vi "Configure Sweep Mode.vi"(5 "Return Time (1s)":dbl=1.0 format="%#.6g", 7 "Hold Time (0 s)":dbl format="%#.6g", 8 "error in (no error)":errorcluster, 9 "Sweep Mode (0: Repeated)":u16(ring) items=["Repeated", "Triggered"], 10 "Channel (0: Channel 1)":u16(ring) items=["Channel 1", "Channel 2"], 11 "VISA resource name":refnum<visa-resource-name>) -> (0 "error out":errorcluster, 3 "VISA resource name out":refnum<visa-resource-name>)   [LabVIEW 2015, in "Tektronix AFG 3000 Series.lvlib"]
doc: "Configures the sweep mode. The VI decides whether the function generator produces a sweep when it receives a trigger or continuous sweep at a rate spedified by sweep time, hold time and return time."
uses:
  Tektronix AFG 3000 Series.lvlib
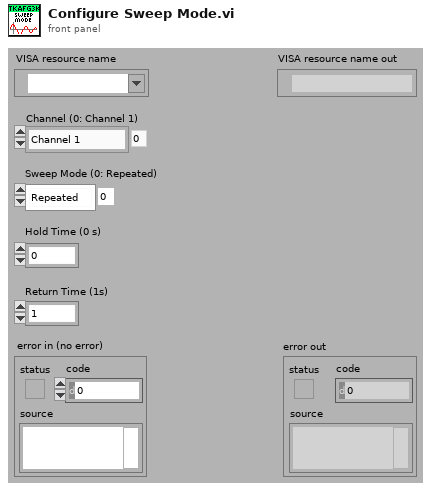
[diagram p1: front panel]
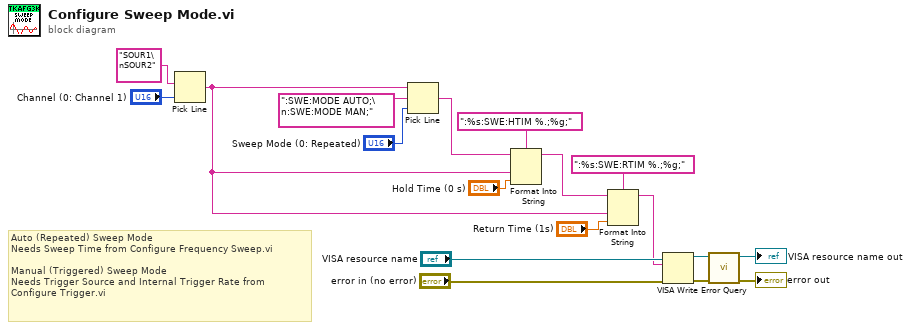
[diagram p0: block diagram]
diagram:
  # "Auto (Repeated) Sweep Mode\nNeeds Sweep Time from Configure Frequency Sweep.vi\n\nManual (Triggered) Sweep Mode\nNeeds Trigger Source and Internal Trigger Rate from\nConfigure Trigger.vi"
  n1 = Pick Line(multi-line string="SOUR1\nSOUR2" ("string (\"\")"), line index="Channel (0: Channel 1)") -> (output string=w2:string)  [unwired: 1 in]
  n2 = Pick Line(string ("")=w2, multi-line string=":SWE:MODE AUTO;\n:SWE:MODE MAN;", line index="Sweep Mode (0: Repeated)") -> (output string=w6:string)
  n3 = Format Into String(format string=":%s:SWE:HTIM %.;%g;", initial string=w6, w2, "Hold Time (0 s)") -> (resulting string=w11:string)  [unwired: 1 in, 1 out]
  n4 = Format Into String(format string=":%s:SWE:RTIM %.;%g;", initial string=w11, w2, "Return Time (1s)") -> (resulting string=w1:string)  [unwired: 1 in, 1 out]
  n5 = VISA Write(VISA resource name="VISA resource name", write buffer=w1, error in (no error)="error in (no error)") -> (VISA resource name out=w14:refnum<visa-resource-name>, error out=w15:errorcluster)  [unwired: 1 out]
  n6 = call "Error Query.vi"("error in (no error)"=w15, "VISA resource name"=w14) -> ("error out"=→"error out":errorcluster, "VISA resource name out"=→"VISA resource name out":refnum<visa-resource-name>)  [unwired: 6 in, 2 out]
